vi "Read Default Image Path.vi"(8 "error in":errorcluster, 10 "Image in":T1, 11 "Config Manager in":refnum<class "Config Manager.lvclass">) -> (0 "error out":errorcluster, 2 "Path out":path, 3 "Config Manager out":refnum<class "Config Manager.lvclass">)   [LabVIEW 2017, in "Config Manager.lvclass"]
uses:
  Config Manager.lvclass
  <vilib>/vision/Image Controls.llb/IMAQ Image.ctl
  Config Manager.lvclass/Config Manager.ctl
  <vilib>/Utility/config.llb/Read Key (String).vi
  <vilib>/Utility/config.llb/NI_LVConfig.lvlib
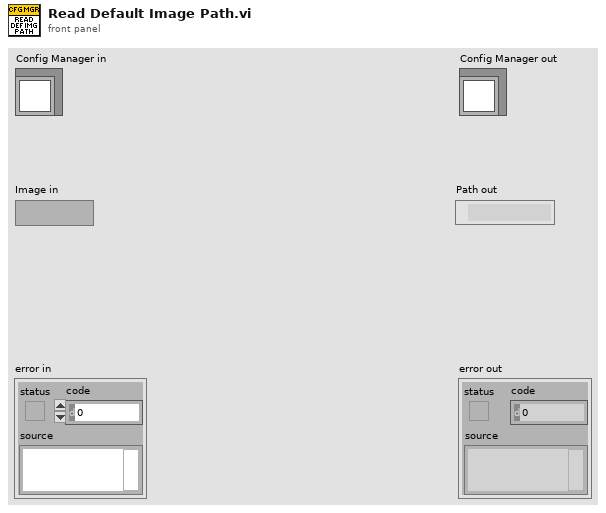
[diagram p1: front panel]
types:
  T1 = typedef "IMAQ Image.ctl" = refnum<image>
  T2 = typedef "NI_LVConfig.lvlib/Config Data RefNum.ctl" = refnum<k1>
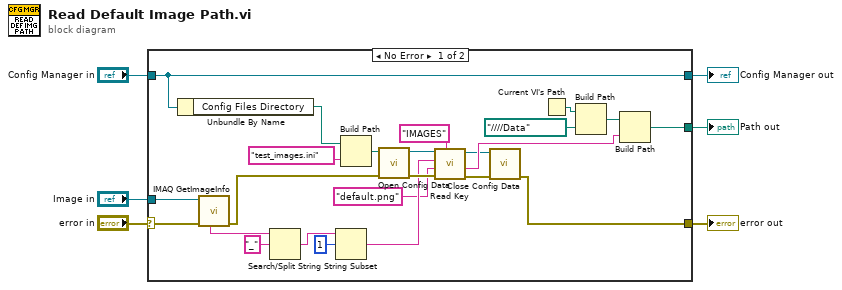
[diagram p0: block diagram]
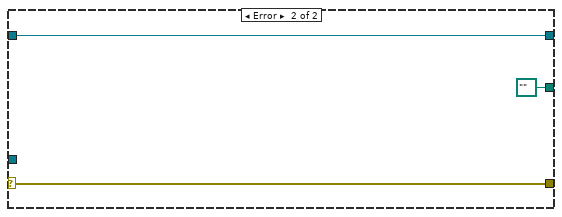
[diagram p2: hidden frame]
diagram:
  n1 = case shown="No Error" "error in" {
    selector: "error in" -> [w9 w33]
    tunnel: [w10 w33] -> w5
    tunnel: [w13 w32] -> w3
    tunnel: "Config Manager in" -> [w13 w32]
    tunnel: "Image in" -> [w14 _]
    tunnel: [w11 path "" ("appended path")] -> w1
    frame No Error {
      n2 = Unbundle By Name(w13) -> ("Config Files Directory"=w12:path)
      n3 = call "IMAQ GetImageInfo"("error in (no error)"=w9, "Image"=w14) -> ("error out"=w8:errorcluster, "Image Name"=w30:string)  [unwired: 2 in, 6 out]
      n4 = Search/Split String(string=w30, search string/char (-)="_") -> (match + rest of string=w28:string)  [unwired: 1 in, 2 out]
      n5 = String Subset(string=w28, offset (0)=1) -> (substring=w19:string)  [unwired: 1 in]
      n6 = Build Path(base path=w12, name or relative path="test_images.ini") -> (appended path=w23:path)
      n7 = call <vilib>:"Open Config Data.vi"("error in (no error)"=w8, "configuration file path"=w23) -> ("error out"=w22:errorcluster, "refnum"=w21:T2)  [unwired: 7 in, 1 out]
      n8 = call-poly <vilib>:"Read Key.vi"("section"="IMAGES", "error in (no error)"=w22, "default value"="default.png", "key"=w19, "refnum"=w21) -> ("error out"=w16:errorcluster, "value"=w17:string, "refnum out"=w15:T2)  [unwired: 3 in, 1 out]
      n9 = call <vilib>:"Close Config Data.vi"("error in (no error)"=w16, "refnum"=w15) -> ("error out"=w10:errorcluster)  [unwired: 8 in, 1 out]
      n10 = Current VI's Path() -> (path=w7:path)
      n11 = Build Path(base path=w7, name or relative path=path "../../../../Data" ("appended path")) -> (appended path=w25:path)
      n12 = Build Path(base path=w25, name or relative path=w17) -> (appended path=w11:path)
    }
    frame Error {
    }
  }
  "error out" <- w5
  "Config Manager out" <- w3
  "Path out" <- w1
